vi "(7) part 2 que.vi"() -> ()   [LabVIEW 2025]
panel:
  out "text":string
  in  "Numeric":u64
  in  "file path (use dialog)":path
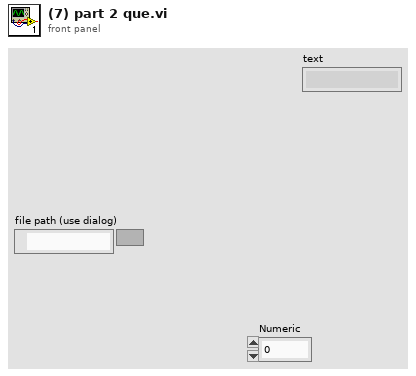
[diagram p1: front panel]
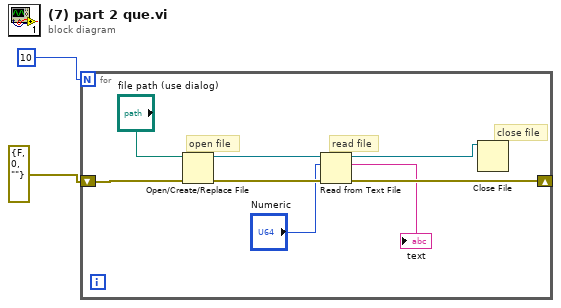
[diagram p0: block diagram]
diagram:
  n1 = for {
    N: 10 -> [_]
    shift-right: [w6] -> _
    shift-left: errorcluster {"status"=FALSE, "code"=0, "source"=""} ("error constant") -> [w9]
    # "open file"
    # "read file"
    # "close file"
    n2 = Open/Create/Replace File(file path (use dialog)="file path (use dialog)", error in=w9) -> (refnum out=w8:refnum<file>, error out=w7:errorcluster)  [unwired: 4 in, 1 out]
    n3 = Read from Text File(file (use dialog)=w8, count="Numeric", error in=w7) -> (refnum out=w5:refnum<file>, text=→"text":string, error out=w6:errorcluster)  [unwired: 1 in, 1 out]
    n4 = Close File(refnum=w5) -> ()  [unwired: 1 in, 2 out]
  }
